vi "stress-test.vi"() -> ()   [LabVIEW 2026]
uses:
  <instrlib>/Keithley 2600 Series/Keithley 2600 Series.lvlib
panel:
  out "appended path 2":path
  out "appended path":path
  in  "nome file 5":string="test-finale-IDVG"
  in  "nome file 4":string="test-finale-IDVD"
  in  "Cluster 7":T1={"numero di sweep ripetute\n(piramidi per dual sweep)"=8, "Delay Time (S)"=0.001, "Numero di punti"=66, "nplc"=0.1, "dual sweep"=FALSE, "autorange source gate"=FALSE, "source_range_gate"=20.0, "String"="0,1,2,3,4,5,6,7", "limit-gate"=1.0, "Source Function Gate"=1, "Range Mode Gate"=0, "range-gate"=1.0, "Autozero Mode Gate"=1, "autorange source drain"=FALSE, "source_range_drain"=20.0, "Pulse Start Level (0 V) 2"=-5.0, "Pulse Stop Level (1 V) 2"=1.5, "limit-drain"=0.001, "Source Function Drain"=1, "Range Mode Drain"=0, "range-drain"=0.001, "Autozero Mode Drain"=1, "inverti smu"=TRUE} {"Autozero Mode Drain" items=["Autozero Off", "Autozero Once", "Autozero Auto"]; "range-drain" items=["100 nA"=1e-07, "1 uA"=1e-06, "10 uA"=1e-05, "100 uA"=0.0001, "1 mA"=0.001, "10 mA"=0.01, "100 mA"=0.1, "1 A"=1.0]; "Range Mode Drain" items=["Auto Range Off", "Auto Range On", "Auto Range Follow Limit"]; "Source Function Drain" items=["Current", "Voltage"]; "limit-drain" format="%#_13g"; "source_range_drain" items=["200 mV"=0.2, "2 V"=2.0, "20 V"=20.0, "200 V"=200.0]; "Autozero Mode Gate" items=["Autozero Off", "Autozero Once", "Autozero Auto"]; "range-gate" items=["100 nA"=1e-07, "1 uA"=1e-06, "10 uA"=1e-05, "100 uA"=0.0001, "1 mA"=0.001, "10 mA"=0.01, "100 mA"=0.1, "1 A"=1.0]; "Range Mode Gate" items=["Auto Range Off", "Auto Range On", "Auto Range Follow Limit"]; "Source Function Gate" items=["Current", "Voltage"]; "limit-gate" format="%#_13g"; "source_range_gate" items=["200 mV"=0.2, "2 V"=2.0, "20 V"=20.0, "200 V"=200.0]; "nplc" items=["0,01"=0.01, "0,1"=0.1, "1"=1.0]}
  in  "Cluster 6":T1={"numero di sweep ripetute\n(piramidi per dual sweep)"=7, "Delay Time (S)"=0.001, "Numero di punti"=71, "nplc"=0.1, "dual sweep"=FALSE, "autorange source gate"=FALSE, "source_range_gate"=20.0, "String"="-5,-4,-3,-2,-1,0,1", "limit-gate"=0.001, "Source Function Gate"=1, "Range Mode Gate"=0, "range-gate"=0.001, "Autozero Mode Gate"=1, "autorange source drain"=FALSE, "source_range_drain"=20.0, "Pulse Start Level (0 V) 2"=0.0, "Pulse Stop Level (1 V) 2"=7.0, "limit-drain"=1.0, "Source Function Drain"=1, "Range Mode Drain"=0, "range-drain"=1.0, "Autozero Mode Drain"=1, "inverti smu"=FALSE} {"Autozero Mode Drain" items=["Autozero Off", "Autozero Once", "Autozero Auto"]; "range-drain" items=["100 nA"=1e-07, "1 uA"=1e-06, "10 uA"=1e-05, "100 uA"=0.0001, "1 mA"=0.001, "10 mA"=0.01, "100 mA"=0.1, "1 A"=1.0]; "Range Mode Drain" items=["Auto Range Off", "Auto Range On", "Auto Range Follow Limit"]; "Source Function Drain" items=["Current", "Voltage"]; "limit-drain" format="%#_13g"; "source_range_drain" items=["200 mV"=0.2, "2 V"=2.0, "20 V"=20.0, "200 V"=200.0]; "Autozero Mode Gate" items=["Autozero Off", "Autozero Once", "Autozero Auto"]; "range-gate" items=["100 nA"=1e-07, "1 uA"=1e-06, "10 uA"=1e-05, "100 uA"=0.0001, "1 mA"=0.001, "10 mA"=0.01, "100 mA"=0.1, "1 A"=1.0]; "Range Mode Gate" items=["Auto Range Off", "Auto Range On", "Auto Range Follow Limit"]; "Source Function Gate" items=["Current", "Voltage"]; "limit-gate" format="%#_13g"; "source_range_gate" items=["200 mV"=0.2, "2 V"=2.0, "20 V"=20.0, "200 V"=200.0]; "nplc" items=["0,01"=0.01, "0,1"=0.1, "1"=1.0]}
  in  "Cluster 5":T1={"numero di sweep ripetute\n(piramidi per dual sweep)"=8, "Delay Time (S)"=0.001, "Numero di punti"=66, "nplc"=0.1, "dual sweep"=FALSE, "autorange source gate"=FALSE, "source_range_gate"=20.0, "String"="0,1,2,3,4,5,6,7", "limit-gate"=1.0, "Source Function Gate"=1, "Range Mode Gate"=0, "range-gate"=1.0, "Autozero Mode Gate"=1, "autorange source drain"=FALSE, "source_range_drain"=20.0, "Pulse Start Level (0 V) 2"=-5.0, "Pulse Stop Level (1 V) 2"=1.5, "limit-drain"=0.001, "Source Function Drain"=1, "Range Mode Drain"=0, "range-drain"=0.001, "Autozero Mode Drain"=1, "inverti smu"=TRUE} {"Autozero Mode Drain" items=["Autozero Off", "Autozero Once", "Autozero Auto"]; "range-drain" items=["100 nA"=1e-07, "1 uA"=1e-06, "10 uA"=1e-05, "100 uA"=0.0001, "1 mA"=0.001, "10 mA"=0.01, "100 mA"=0.1, "1 A"=1.0]; "Range Mode Drain" items=["Auto Range Off", "Auto Range On", "Auto Range Follow Limit"]; "Source Function Drain" items=["Current", "Voltage"]; "limit-drain" format="%#_13g"; "source_range_drain" items=["200 mV"=0.2, "2 V"=2.0, "20 V"=20.0, "200 V"=200.0]; "Autozero Mode Gate" items=["Autozero Off", "Autozero Once", "Autozero Auto"]; "range-gate" items=["100 nA"=1e-07, "1 uA"=1e-06, "10 uA"=1e-05, "100 uA"=0.0001, "1 mA"=0.001, "10 mA"=0.01, "100 mA"=0.1, "1 A"=1.0]; "Range Mode Gate" items=["Auto Range Off", "Auto Range On", "Auto Range Follow Limit"]; "Source Function Gate" items=["Current", "Voltage"]; "limit-gate" format="%#_13g"; "source_range_gate" items=["200 mV"=0.2, "2 V"=2.0, "20 V"=20.0, "200 V"=200.0]; "nplc" items=["0,01"=0.01, "0,1"=0.1, "1"=1.0]}
  in  "nome file 3":string="test-iniziale-IDVG-ciclo"
  out "path 3":path
  in  "Cluster 4":T1={"numero di sweep ripetute\n(piramidi per dual sweep)"=7, "Delay Time (S)"=0.001, "Numero di punti"=71, "nplc"=0.1, "dual sweep"=FALSE, "autorange source gate"=FALSE, "source_range_gate"=20.0, "String"="-5,-4,-3,-2,-1,0,1", "limit-gate"=0.001, "Source Function Gate"=1, "Range Mode Gate"=0, "range-gate"=0.001, "Autozero Mode Gate"=1, "autorange source drain"=FALSE, "source_range_drain"=20.0, "Pulse Start Level (0 V) 2"=0.0, "Pulse Stop Level (1 V) 2"=7.0, "limit-drain"=1.0, "Source Function Drain"=1, "Range Mode Drain"=0, "range-drain"=1.0, "Autozero Mode Drain"=1, "inverti smu"=FALSE} {"Autozero Mode Drain" items=["Autozero Off", "Autozero Once", "Autozero Auto"]; "range-drain" items=["100 nA"=1e-07, "1 uA"=1e-06, "10 uA"=1e-05, "100 uA"=0.0001, "1 mA"=0.001, "10 mA"=0.01, "100 mA"=0.1, "1 A"=1.0]; "Range Mode Drain" items=["Auto Range Off", "Auto Range On", "Auto Range Follow Limit"]; "Source Function Drain" items=["Current", "Voltage"]; "limit-drain" format="%#_13g"; "source_range_drain" items=["200 mV"=0.2, "2 V"=2.0, "20 V"=20.0, "200 V"=200.0]; "Autozero Mode Gate" items=["Autozero Off", "Autozero Once", "Autozero Auto"]; "range-gate" items=["100 nA"=1e-07, "1 uA"=1e-06, "10 uA"=1e-05, "100 uA"=0.0001, "1 mA"=0.001, "10 mA"=0.01, "100 mA"=0.1, "1 A"=1.0]; "Range Mode Gate" items=["Auto Range Off", "Auto Range On", "Auto Range Follow Limit"]; "Source Function Gate" items=["Current", "Voltage"]; "limit-gate" format="%#_13g"; "source_range_gate" items=["200 mV"=0.2, "2 V"=2.0, "20 V"=20.0, "200 V"=200.0]; "nplc" items=["0,01"=0.01, "0,1"=0.1, "1"=1.0]}
  in  "base path 2":path=path "C:/Users/gioel/Koofr/università/tesi_magistrale/misure/stress-test"
  in  "nome file 2":string="test-iniziale-IDVD-ciclo"
  out "path 2":path
  in  "tensione di stress drain":dbl[](array[numeric])=[10.0, 20.0, 30.0, 40.0, 50.0, 60.0, 70.0, 80.0, 90.0, 100.0]
  in  "Cluster":T2={"Numero di punti"=60, "fattore-measdelay"=65, "Periodo"=1.0, "source autorange gate"=FALSE, "Tensione gate"=-5.0, "llimit-gate"=0.001, "Source Function Gate"=1, "Range Mode Gate"=0, "Autozero Mode Gate"=1, "tensione drain"=1.0, "limit-drain"=0.001, "Autozero Mode Drain"=1, "Source Function Drain"=1, "Range Mode Drain"=0, "source autorange drain"=FALSE, "range-gate"=0.001, "source_range_gate"=20.0, "range-drain"=0.001, "source_range_drain"=200.0} {"source_range_drain" items=["200 mV"=0.2, "2 V"=2.0, "20 V"=20.0, "200 V"=200.0]; "range-drain" items=["100 nA"=1e-07, "1 uA"=1e-06, "10 uA"=1e-05, "100 uA"=0.0001, "1 mA"=0.001, "10 mA"=0.01, "100 mA"=0.1, "1 A"=1.0]; "source_range_gate" items=["200 mV"=0.2, "2 V"=2.0, "20 V"=20.0, "200 V"=200.0]; "range-gate" items=["100 nA"=1e-07, "1 uA"=1e-06, "10 uA"=1e-05, "100 uA"=0.0001, "1 mA"=0.001, "10 mA"=0.01, "100 mA"=0.1, "1 A"=1.0]; "Range Mode Drain" items=["Auto Range Off", "Auto Range On", "Auto Range Follow Limit"]; "Source Function Drain" items=["Current", "Voltage"]; "Autozero Mode Drain" items=["Autozero Off", "Autozero Once", "Autozero Auto"]; "limit-drain" format="%#_13g"; "Autozero Mode Gate" items=["Autozero Off", "Autozero Once", "Autozero Auto"]; "Range Mode Gate" items=["Auto Range Off", "Auto Range On", "Auto Range Follow Limit"]; "Source Function Gate" items=["Current", "Voltage"]; "llimit-gate" format="%#_13g"; "Periodo" items=["500 uS", "1 mS", "2 mS", "5 mS", "10 mS", "20 mS", "50 mS", "100 mS", "200 mS", "500 mS", "1 S", "2 S", "5 S", "10 S", ""]}
  in  "Misura":bool
  in  "stop 2":bool
  in  "Numero Cicli":i32=10
  in  "nome file":string="stress_ciclo"
  out "path":path
  out "ciclo attuale":i32
  out "error out":errorcluster
  in  "stop":bool
  out "Firmware Revision":string
  out "Serial Number":string
  out "Model":string
  in  "VISA resource name":refnum<visa-resource-name>="USB0::0x05E6::0x2612::4671051::INSTR"
  # "Impostazioni connessione"
  # "Impostazioni comuni"
  # "tabella valori"
  # "Controllo misura"
  # "TENSIONE DI STRESS\nDRAIN"
  # "USARE QUESTO"
  # "tensione drain nei comandi bias non è abilitato"
  # "Impostazioni comuni"
  # "Impostazioni funzione source"
  # "DRAIN"
  # "GATE"
  # "Controllo misura"
  # "non utilizzato...funzioni di lua per automatizzare il range"
  # "Impostazioni funzione misura"
  # "DRAIN"
  # "GATE"
  # "Impostazioni comuni"
  # "Impostazioni funzione source"
  # "DRAIN"
  # "GATE"
  # "Controllo misura"
  # "non utilizzato...funzioni di lua per automatizzare il range"
  # "Impostazioni funzione misura"
  # "DRAIN"
  # "GATE"
  # "Impostazioni comuni"
  # "Impostazioni funzione source"
  # "DRAIN"
  # "GATE"
  # "Controllo misura"
  # "non utilizzato...funzioni di lua per automatizzare il range"
  # "Impostazioni funzione misura"
  # "DRAIN"
  # "GATE"
  # "Impostazioni comuni"
  # "Impostazioni funzione source"
  # "DRAIN"
  # "GATE"
  # "Controllo misura"
  # "non utilizzato...funzioni di lua per automatizzare il range"
  # "Impostazioni funzione misura"
  # "DRAIN"
  # "GATE"
  # "Impostazioni comuni"
  # "Impostazioni funzione source"
  # "GATE"
  # "DRAIN"
  # "Controllo misura"
  # "NON ABILITATO"
  # "Impostazioni funzione misura"
  # "GATE"
  # "DRAIN"
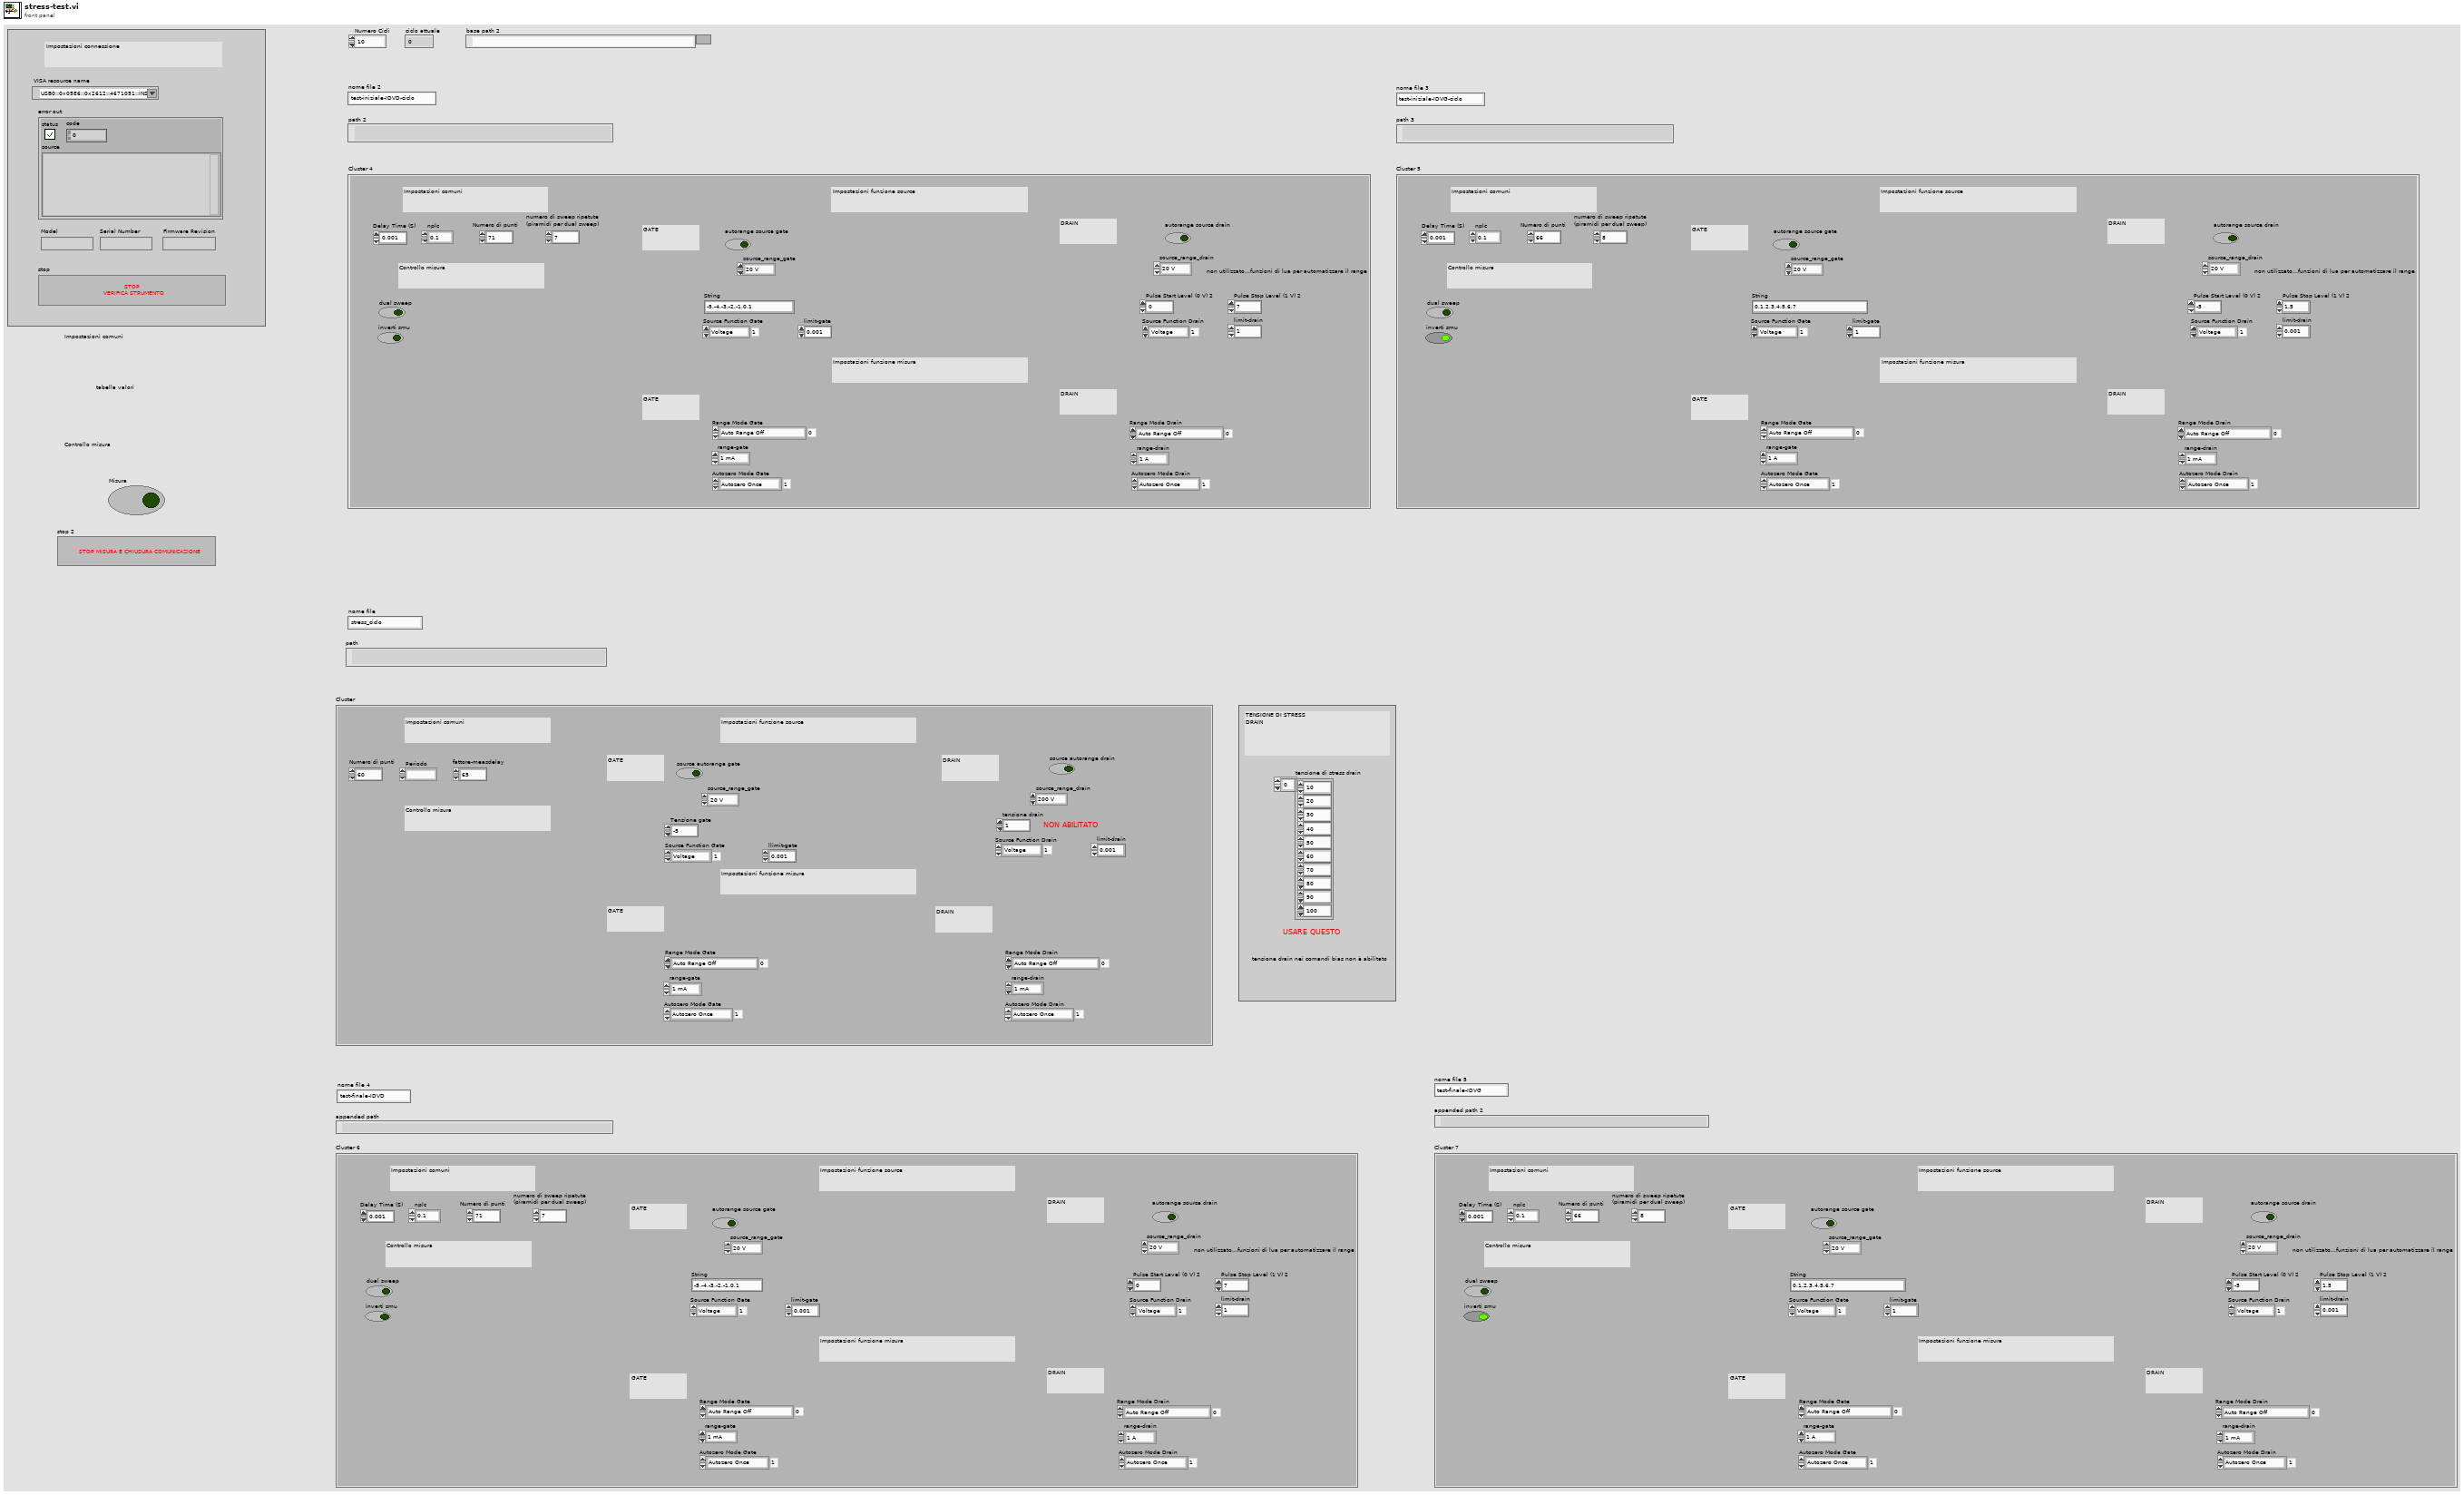
[diagram p1: front panel]
types:
  T1 = cluster{"numero di sweep ripetute\n(piramidi per dual sweep)":i32, "Delay Time (S)":dbl, "Numero di punti":i32, "nplc":dbl, "dual sweep":bool, "autorange source gate":bool, "source_range_gate":dbl, "String":string, "limit-gate":dbl, "Source Function Gate":i32, "Range Mode Gate":i32, "range-gate":dbl, "Autozero Mode Gate":i32, "autorange source drain":bool, "source_range_drain":dbl, "Pulse Start Level (0 V) 2":dbl, "Pulse Stop Level (1 V) 2":dbl, "limit-drain":dbl, "Source Function Drain":i32, "Range Mode Drain":i32, "range-drain":dbl, "Autozero Mode Drain":i32, "inverti smu":bool}
  T2 = cluster{"Numero di punti":i32, "fattore-measdelay":i32, "Periodo":ext, "source autorange gate":bool, "Tensione gate":dbl, "llimit-gate":dbl, "Source Function Gate":i32, "Range Mode Gate":i32, "Autozero Mode Gate":i32, "tensione drain":dbl, "limit-drain":dbl, "Autozero Mode Drain":i32, "Source Function Drain":i32, "Range Mode Drain":i32, "source autorange drain":bool, "range-gate":dbl, "source_range_gate":dbl, "range-drain":dbl, "source_range_drain":dbl}
  T3 = cluster{"VISA resource name out":refnum<visa-resource-name>, "error out":errorcluster}
  T4 = cluster{"SMUA-CORRENTE":dbl[], "SMUA-TENSIONE":dbl[], "SMUA-TEMPI":dbl[], "SMUB-CORRENTE":dbl[], "SMUB-TENSIONE":dbl[], "SMUB-TEMPI":dbl[]}
  T5 = cluster{"CORRENTE SMUA":dbl[], "TENSIONE SMUA":dbl[], "TEMPI SMUA":dbl[], "CORRENTE 2":dbl[], "TENSIONE 2":dbl[], "TEMPI 2":dbl[]}
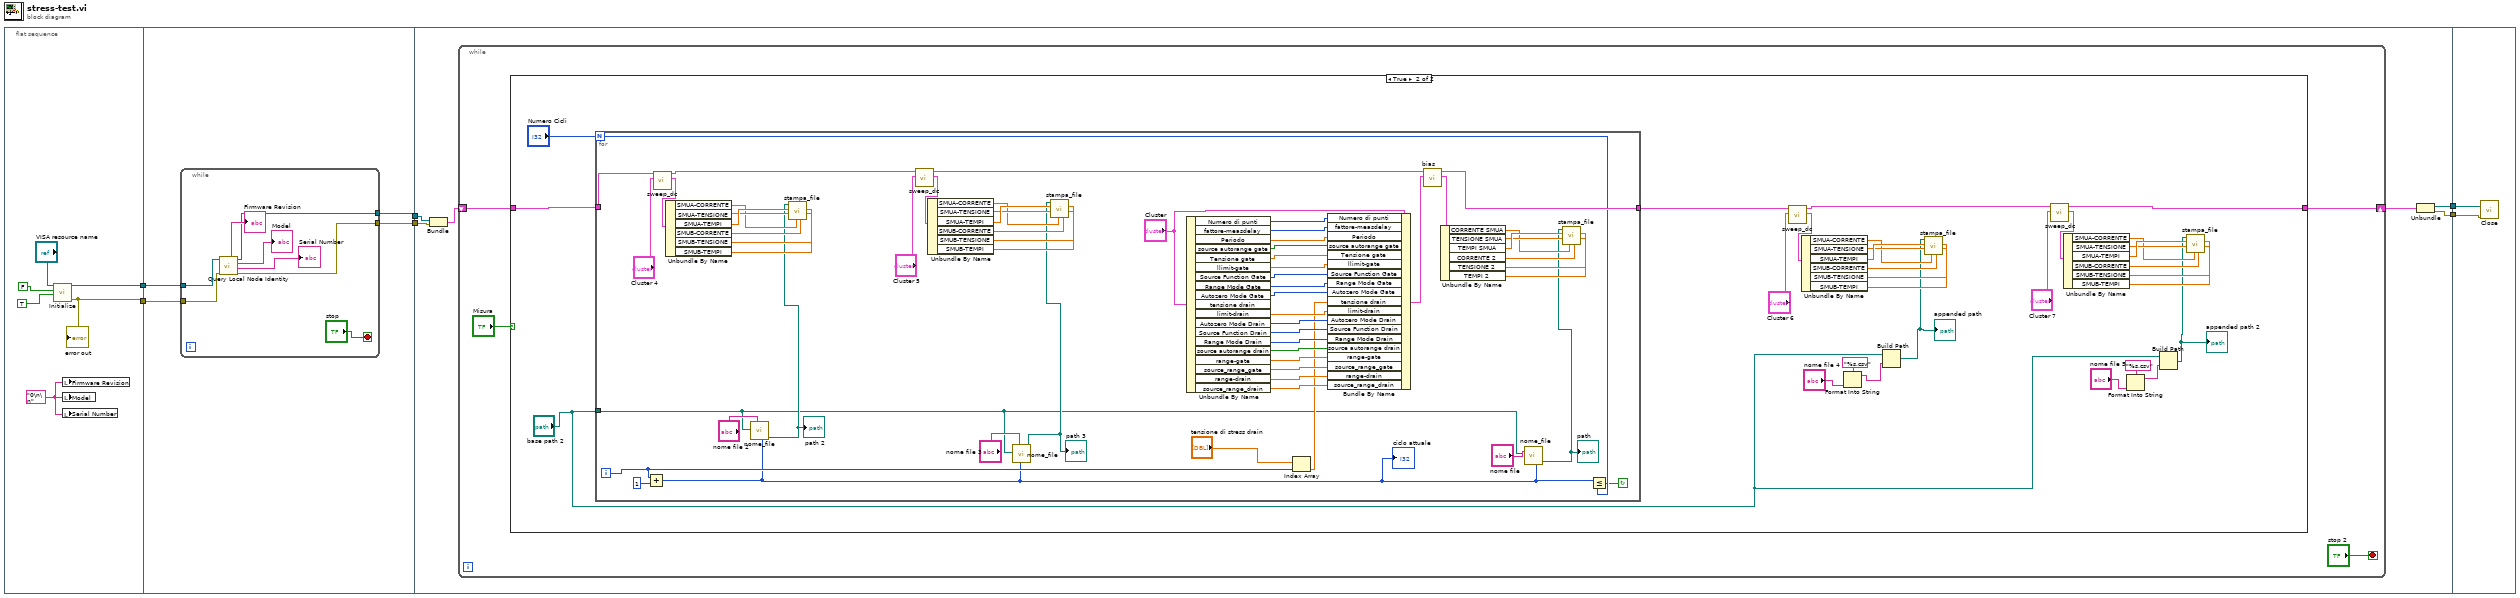
[diagram p0: block diagram]
diagram:
  n1 = flat-sequence {
    tunnel: [w10] -> w5
    tunnel: [w7] -> w4
    tunnel: [w14] -> w6
    tunnel: w5 -> [w16]
    tunnel: w4 -> [w15]
    tunnel: [w13] -> w3
    tunnel: w6 -> [w30]
    tunnel: w3 -> [w29]
    tunnel: [w26] -> w2
    tunnel: [w25] -> w1
    tunnel: w2 -> [w128]
    tunnel: w1 -> [w127]
    frame #0 {
      w11 = "0\n\n"
      n2 = call <instrlib>:"Initialize.vi"("Reset (True)"=TRUE, "ID Query (True)"=FALSE, "VISA resource name"="VISA resource name") -> ("error out"=w7:errorcluster, "VISA resource name out"=w10:refnum<visa-resource-name>)  [unwired: 7 in]
      "error out" <- w7
      n3 = local write "Firmware Revision"(w11) -> ()
      n4 = local write "Model"(w11) -> ()
      n5 = local write "Serial Number"(w11) -> ()
    }
    frame #1 {
      n6 = while {
        tunnel: w16 -> [w20]
        tunnel: w15 -> [w19]
        tunnel: [w18] -> w14
        tunnel: [w17] -> w13
        stop <- "stop" stop-if-true
        n7 = call <instrlib>:"Query Local Node Identity.vi"("error in (no error)"=w19, "VISA resource name"=w20) -> ("error out"=w17:errorcluster, "Serial Number"=→"Serial Number":string, "Model"=→"Model":string, "VISA resource name out"=w18:refnum<visa-resource-name>, "Firmware Revision"=→"Firmware Revision":string)  [unwired: 5 in]
      }
    }
    frame #2 {
      n8 = Bundle("VISA resource name out"=w30, "error out"=w29) -> (w28:T3)  [unwired: 1 in]
      n9 = while {
        shift-right: [w34] -> w27
        shift-left: w28 -> [w31]
        stop <- "stop 2" stop-if-true
        n10 = case shown="True" "Misura" {
          tunnel: w31 -> [w35 w64]
          tunnel: [w35 w45] -> w34
          frame False {
          }
          frame True {
            n11 = for {
              N: "Numero Cicli" -> [w115]
              tunnel: [w126] -> w46
              tunnel: w64 -> [w92]
              tunnel: "base path 2" -> [w67]
              i -> [w93]
              stop <- w68 continue-if-true
              n12 = Add(x=w93, y=1) -> (x+y=w71:i32)
              "ciclo attuale" <- w71
              n13 = call "sweep_dc.vi"("Cluster 4"="Cluster 4", "Cluster"=w92) -> ("Cluster 3"=w83:T4, "Cluster 2"=w70:T3)  [unwired: 8 in]
              n14 = Unbundle By Name(w83) -> ("SMUA-CORRENTE"=w89:dbl[], "SMUA-TENSIONE"=w90:dbl[], "SMUA-TEMPI"=w91:dbl[], "SMUB-CORRENTE"=w87:dbl[], "SMUB-TENSIONE"=w86:dbl[], "SMUB-TEMPI"=w88:dbl[])
              n15 = call "nome_file.vi"("numero file"=w71, "nome file"="nome file 2", "percorso iniziale"=w67) -> ("risulato percorso"=w84:path)  [unwired: 8 in]
              "path 2" <- w84
              n16 = call "stampa_file.vi"(1:"Tensione"=w86, 2:"Tempo"=w88, 4:"Corrente"=w87, 6:"Corrente"=w89, 9:"Tensione"=w90, 10:"Tempo"=w91, "file path (dialog if empty)"=w84) -> ()  [unwired: 3 in, 2 out]
              n17 = call "sweep_dc.vi"("Cluster 4"="Cluster 5", "Cluster"=w70) -> ("Cluster 3"=w73:T4, "Cluster 2"=w69:T3)  [unwired: 8 in]
              n18 = Unbundle By Name(w73) -> ("SMUA-CORRENTE"=w79:dbl[], "SMUA-TENSIONE"=w80:dbl[], "SMUA-TEMPI"=w81:dbl[], "SMUB-CORRENTE"=w77:dbl[], "SMUB-TENSIONE"=w76:dbl[], "SMUB-TEMPI"=w78:dbl[])
              n19 = call "nome_file.vi"("numero file"=w71, "nome file"="nome file 3", "percorso iniziale"=w67) -> ("risulato percorso"=w74:path)  [unwired: 8 in]
              "path 3" <- w74
              n20 = call "stampa_file.vi"(1:"Tensione"=w76, 2:"Tempo"=w78, 4:"Corrente"=w77, 6:"Corrente"=w79, 9:"Tensione"=w80, 10:"Tempo"=w81, "file path (dialog if empty)"=w74) -> ()  [unwired: 3 in, 2 out]
              n21 = Unbundle By Name("Cluster") -> ("Numero di punti"=w112:i32, "fattore-measdelay"=w111:i32, "Periodo"=w110:ext, "source autorange gate"=w109:bool, "Tensione gate"=w108:dbl, "llimit-gate"=w107:dbl, "Source Function Gate"=w106:i32, "Range Mode Gate"=w105:i32, "Autozero Mode Gate"=w104:i32, "limit-drain"=w103:dbl, "Autozero Mode Drain"=w102:i32, "Source Function Drain"=w101:i32, "Range Mode Drain"=w100:i32, "source autorange drain"=w99:bool, "range-gate"=w98:dbl, "source_range_gate"=w97:dbl, "range-drain"=w96:dbl, "source_range_drain"=w95:dbl)  [unwired: 1 out]
              n22 = Index Array(array="tensione di stress drain", index=w93) -> (element=w94:dbl)
              n23 = Bundle By Name(cluster="Cluster", "Numero di punti"=w112, "fattore-measdelay"=w111, "Periodo"=w110, "source autorange gate"=w109, "Tensione gate"=w108, "llimit-gate"=w107, "Source Function Gate"=w106, "Range Mode Gate"=w105, "Autozero Mode Gate"=w104, "tensione drain"=w94, "limit-drain"=w103, "Autozero Mode Drain"=w102, "Source Function Drain"=w101, "Range Mode Drain"=w100, "source autorange drain"=w99, "range-gate"=w98, "source_range_gate"=w97, "range-drain"=w96, "source_range_drain"=w95) -> (w114:T2)
              n24 = call "bias.vi"("Cluster"=w114, "Cluster 3"=w69) -> ("Cluster 2"=w125:T5, "output cluster"=w126:T3)  [unwired: 8 in]
              n25 = Unbundle By Name(w125) -> ("CORRENTE SMUA"=w122:dbl[], "TENSIONE SMUA"=w123:dbl[], "TEMPI SMUA"=w124:dbl[], "CORRENTE 2"=w120:dbl[], "TENSIONE 2"=w119:dbl[], "TEMPI 2"=w121:dbl[])
              n26 = call "nome_file.vi"("numero file"=w71, "nome file"="nome file", "percorso iniziale"=w67) -> ("risulato percorso"=w116:path)  [unwired: 8 in]
              "path" <- w116
              n27 = call "stampa_file.vi"(1:"Tensione"=w119, 2:"Tempo"=w121, 4:"Corrente"=w120, 6:"Corrente"=w122, 9:"Tensione"=w123, 10:"Tempo"=w124, "file path (dialog if empty)"=w116) -> ()  [unwired: 3 in, 2 out]
              n28 = Less Or Equal?(x=w71, y=w115) -> (x <= y?=w68:bool)
            }
            n29 = call "sweep_dc.vi"("Cluster 4"="Cluster 6", "Cluster"=w46) -> ("Cluster 3"=w57:T4, "Cluster 2"=w47:T3)  [unwired: 8 in]
            n30 = Unbundle By Name(w57) -> ("SMUA-CORRENTE"=w61:dbl[], "SMUA-TENSIONE"=w62:dbl[], "SMUA-TEMPI"=w63:dbl[], "SMUB-CORRENTE"=w59:dbl[], "SMUB-TENSIONE"=w58:dbl[], "SMUB-TEMPI"=w60:dbl[])
            n31 = Format Into String(format string="%s.csv", "nome file 4") -> (resulting string=w39:string)  [unwired: 2 in, 1 out]
            n32 = Build Path(base path="base path 2", name or relative path=w39) -> (appended path=w43:path)
            "appended path" <- w43
            n33 = call "stampa_file.vi"(1:"Tensione"=w58, 2:"Tempo"=w60, 4:"Corrente"=w59, 6:"Corrente"=w61, 9:"Tensione"=w62, 10:"Tempo"=w63, "file path (dialog if empty)"=w43) -> ()  [unwired: 3 in, 2 out]
            n34 = call "sweep_dc.vi"("Cluster 4"="Cluster 7", "Cluster"=w47) -> ("Cluster 3"=w49:T4, "Cluster 2"=w45:T3)  [unwired: 8 in]
            n35 = Unbundle By Name(w49) -> ("SMUA-CORRENTE"=w53:dbl[], "SMUA-TENSIONE"=w54:dbl[], "SMUA-TEMPI"=w55:dbl[], "SMUB-CORRENTE"=w51:dbl[], "SMUB-TENSIONE"=w50:dbl[], "SMUB-TEMPI"=w52:dbl[])
            n36 = Format Into String(format string="%s.csv", "nome file 5") -> (resulting string=w37:string)  [unwired: 2 in, 1 out]
            n37 = Build Path(base path="base path 2", name or relative path=w37) -> (appended path=w42:path)
            "appended path 2" <- w42
            n38 = call "stampa_file.vi"(1:"Tensione"=w50, 2:"Tempo"=w52, 4:"Corrente"=w51, 6:"Corrente"=w53, 9:"Tensione"=w54, 10:"Tempo"=w55, "file path (dialog if empty)"=w42) -> ()  [unwired: 3 in, 2 out]
          }
        }
      }
      n39 = Unbundle(w27) -> ("VISA resource name out"=w26:refnum<visa-resource-name>, "error out"=w25:errorcluster)
    }
    frame #3 {
      n40 = call <instrlib>:"Close.vi"("error in (no error)"=w127, "VISA resource name"=w128) -> ()  [unwired: 9 in, 1 out]
    }
  }
